vi "Tach_Power_AutoStop.vi"() -> ()   [LabVIEW 2020]
uses:
  <vilib>/Utility/error.llb/DialogType.ctl
  <extravilib>/ChannelInstances/Tag-bool/Read With Abort.vi
  <extravilib>/ChannelInstances/Tag-bool/Write With Abort.vi
  <extravilib>/ChannelInstances/Tag-bool/Instantiate.vi
  <extravilib>/ChannelInstances/Tag-bool/EndpointRead.vi
  <vilib>/Waveform/DWDTOps.llb/DWDT Digital to Analog.vi
  <extravilib>/ChannelInstances/Tag-bool/Endpoint.vi
  <extravilib>/ChannelInstances/Tag-bool.lvlib
panel:
  out "Torque/Power Graph":dynamicdata(graph)
  out "Tach Graph":digitalwaveform[](graph)
  in  "stop":bool
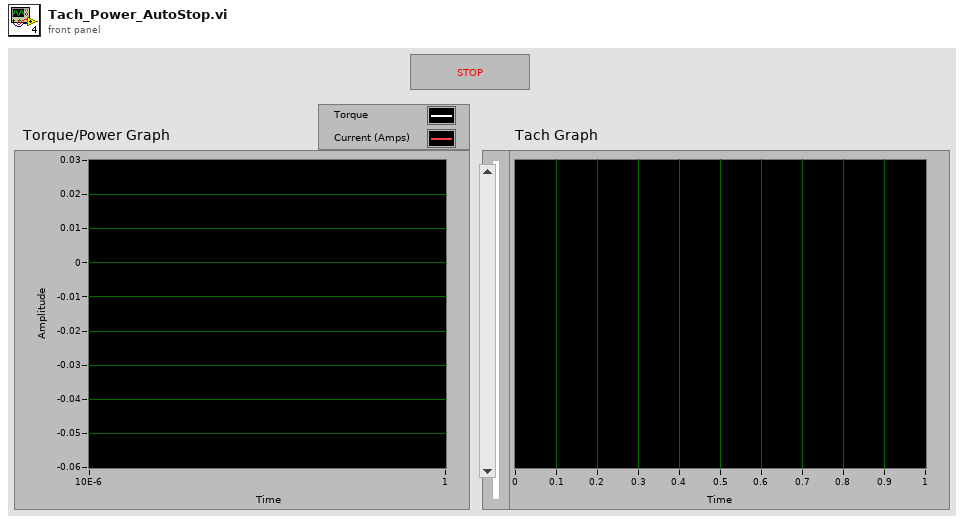
[diagram p1: front panel]
types:
  T1 = typedef "DialogType.ctl" = u16
  T2 = typedef "Tag-bool.lvlib/))Channel.ctl" = refnum<queue>
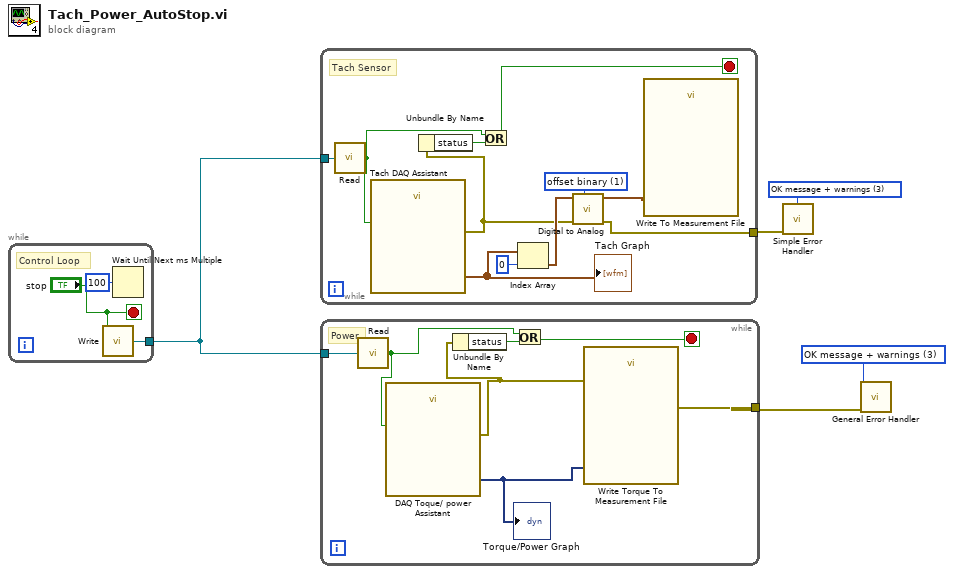
[diagram p0: block diagram]
diagram:
  w2 = T1 3 items=["no dialog", "OK message", "continue or stop message", "OK message + warnings", "continue/stop + warnings"] ("type of dialog (OK msg:1)")
  w5 = T1 3 items=["no dialog", "OK message", "continue or stop message", "OK message + warnings", "continue/stop + warnings"] ("type of dialog (OK msg:1)")
  n1 = while {
    tunnel: [w6] -> w1
    stop <- "stop" stop-if-true
    # "Control Loop"
    n2 = call <extravilib>:"Write.vi"("element"="stop") -> ("channel"=w6:T2)  [unwired: 1 out]
    n3 = Wait Until Next ms Multiple(millisecond multiple=u32 100 ("millisecond timer value")) -> ()  [unwired: 1 out]
  }
  n4 = while {
    tunnel: w1 -> [w19]
    tunnel: [w10] -> w4
    stop <- w18 stop-if-true
    w12 = u16 1 items=["unsigned binary", "offset binary", "2's complement"] ("data format (offset binary)")
    # "Tach Sensor"
    n5 = call <extravilib>:"Read.vi"("channel"=w19) -> ("element"=w16:bool)  [unwired: 1 in, 1 out]
    n6 = call "Tach DAQ Assistant"("stop (F)"=w16) -> ("data"=w15:digitalwaveform[], "error out"=w11:errorcluster)  [unwired: 15 in, 2 out]
    "Tach Graph" <- w15
    n7 = Unbundle By Name(w11) -> ("status"=w17:bool)
    n8 = Or(x=w16, y=w17) -> (x .or. y?=w18:bool)
    n9 = Index Array(array=w15, index=0) -> (element=w13:digitalwaveform)
    n10 = call-poly <vilib>:"Digital to Analog.vi"("data format (offset binary)"=w12, "error in (no error)"=w11, "digital waveform"=w13) -> ("error out"=w10:errorcluster, "analog waveform"=w9:waveform(dbl))  [unwired: 5 in, 2 out]
    n11 = call "Write To Measurement File"("Signals"=w9) -> ()  [unwired: 16 in, 3 out]
  }
  n12 = while {
    tunnel: w1 -> [w26]
    tunnel: [w20] -> w3
    stop <- w24 stop-if-true
    # "Power"
    n13 = call <extravilib>:"Read.vi"("channel"=w26) -> ("element"=w23:bool)  [unwired: 1 in, 1 out]
    n14 = call "DAQ Toque/ power Assistant"("stop (F)"=w23) -> ("data"=w21:dynamicdata, "error out"=w22:errorcluster)  [unwired: 15 in, 2 out]
    "Torque/Power Graph" <- w21
    n15 = Unbundle By Name(w22) -> ("status"=w25:bool)
    n16 = Or(x=w23, y=w25) -> (x .or. y?=w24:bool)
    n17 = call "Write Torque To Measurement File"("Signals"=w21, "error in (no error)"=w22) -> ("error out"=w20:errorcluster)  [unwired: 15 in, 2 out]
  }
  n18 = call <vilib>:"Simple Error Handler.vi"("type of dialog (OK msg:1)"=w5, "error in (no error)"=w4) -> ()  [unwired: 3 in, 5 out]
  n19 = call <vilib>:"General Error Handler.vi"("type of dialog (OK msg:1)"=w2, "error in (no error)"=w3) -> ()  [unwired: 9 in, 5 out]
